vi "Possible Ragged Array.vi"(9 "Array":variant[](array[variant])) -> (3 "Ragged Array posible":bool)   [LabVIEW 2017, in "JSONtext.lvlib"]
uses:
  JSONtext.lvlib
  JSON Value Type.ctl
  <vilib>/Utility/Data Type/Type Definitions/Data Type.ctl
  <vilib>/Utility/Data Type/NI_Data Type.lvlib
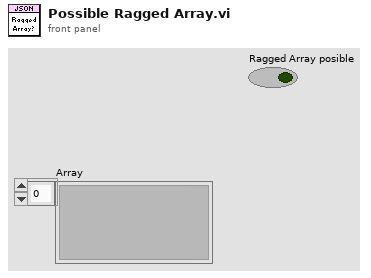
[diagram p1: front panel]
types:
  T1 = typedef "NI_Data Type.lvlib/Data Type.ctl" = enum8{"Invalid Type", "Void", "I8", "I16", "I32", "I64", "U8", "U16", "U32", "U64", "Single Float", "Double Float", "Extended Float", "Single Complex", "Double Complex", "Extended Complex", "Enum U8", "Enum U16", "Enum U32", "Enum U64", "Single Float With Unit", "Double Float With Unit", "Extended Float With Unit", "Single Complex with Unit", "Double Complex with Unit", "Extended Complex with Unit", "Boolean", "String", "Path", "Picture", "Tag", "Array", "Cluster", "Variant", "LV Variant", "Waveform", "Timestamp", "Digital Waveform", "Digital Data", "ExpressData", "Refnum", "External Data", "VI", "Poly VI", "LabVIEW Class Instance", "Fixed Point"}
  T2 = typedef "JSONtext.lvlib/JSON Value Type.ctl" = enum16{"Not a JSON Value", "JSON Object", "JSON Array", "String", "Number", "true", "false", "null"}
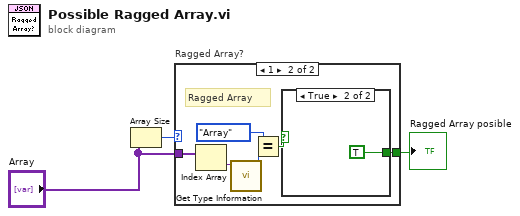
[diagram p0: block diagram]
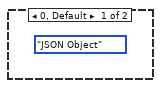
[diagram p2: hidden frame]
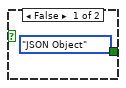
[diagram p3: hidden frame]
diagram:
  n1 = Array Size(array="Array") -> (size(s)=w1:i32)
  n2 = case "Ragged Array?" shown="1" w1 {
    tunnel: "Array" -> [_ w9]
    tunnel: [_ w4] -> w3
    frame 0, Default {
      (unwired) JSON_Value_Type."JSON Object" ("JSON Value Type")
    }
    frame 1 {
      # "Ragged Array"
      n3 = Index Array(array=w9) -> (element=w8:variant)  [unwired: 1 in]
      n4 = call <vilib>:"Get Type Information.vi"("Variant"=w8) -> ("Type"=w7:T1)  [unwired: 6 in, 4 out]
      n5 = Equal?(x=Data_Type."Array", y=w7) -> (x = y?=w5:bool)
      n6 = case shown="True" w5 {
        tunnel: [_ TRUE] -> w4
        frame False {
          (unwired) JSON_Value_Type."JSON Object" ("JSON Value Type")
        }
        frame True {
        }
      }
    }
  }
  "Ragged Array posible" <- w3
